vi "Transceiver.Command.Receive.vi"(8 "error in (no error)":errorcluster, 9 "timeout in ms (0)":i32 format="%d ms", 11 "Transceiver Thread in":refnum<class "Transceiver Thread.lvclass">) -> (0 "error out":errorcluster, 1 "timed out?":bool, 2 "command":T1={"Command"=enum."Rx", "Command Parameters"={"arg1"=0, "arg2"=0}}, 3 "Transceiver Thread out":refnum<class "Transceiver Thread.lvclass">)   [LabVIEW 2017, in "DSF Core.lvlib" / "Transceiver Thread.lvclass"]
uses:
  Transceiver Thread.lvclass
  Interface/Transceiver Interface.Command Data.ctl
  Interface/Transceiver Interface.Command.ctl
  Interface/Transceiver Interface.Command Parameters.ctl
  Transceiver Thread.lvclass/Transceiver Thread.ctl
  Interface/Interface.lvclass/Interface.ctl
  Debug/FIFO Flags.lvclass/FIFO Flags.ctl
  Interface/Transceiver Interface.Read.Command.vi
  Interface/Interface.Read.Command.vi
  Interface/Interface.Get Command FIFO.vi
  Interface/Interface.Get Debug Flags.vi
  Interface/Interface.RT FIFO.Read.16B.vi
  Debug/FIFO Flags.Get Infinite Timeouts.vi
  Interface/Transceiver Interface.lvclass
  C:/Git/DSF/dsf core/Source/Engine/Classes/Interface/Interface.lvclass
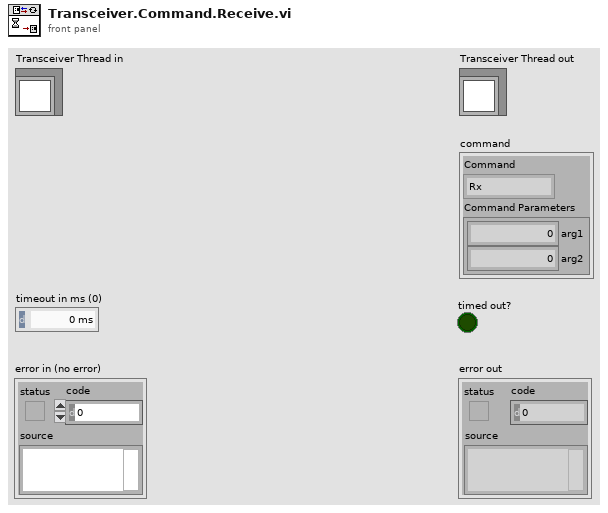
[diagram p1: front panel]
types:
  T1 = typedef "DSF Core.lvlib/Transceiver Interface.lvclass/Transceiver Interface.Command Data.ctl" = cluster{"Command":T2, "Command Parameters":T3}
  T2 = typedef "DSF Core.lvlib/Transceiver Interface.lvclass/Transceiver Interface.Command.ctl" = enum8{"Set Base Pointer", "Rx", "Tx", "Shutdown"}
  T3 = typedef "DSF Core.lvlib/Transceiver Interface.lvclass/Transceiver Interface.Command Parameters.ctl" = cluster{"arg1":u64, "arg2":u64}
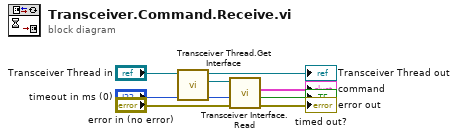
[diagram p0: block diagram]
diagram:
  n1 = call "Transceiver Thread.Get Interface.vi"("Transceiver Thread in"="Transceiver Thread in") -> ("Interface"=w7:refnum<class "Transceiver Interface.lvclass">, "Transceiver Thread out"=→"Transceiver Thread out":refnum<class "Transceiver Thread.lvclass">)  [unwired: 9 in]
  n2 = call-poly "Transceiver Interface.Read.vi"("error in (no error)"="error in (no error)", "timeout in ms (0)"="timeout in ms (0)", "Transceiver Interface in"=w7) -> ("error out"=→"error out":errorcluster, "empty?"=→"timed out?":bool, "command"=→"command":T1)  [unwired: 4 in, 2 out]
